vi "GetTextPositions.vi"(0 "reference":refnum<class "AbstractEdge.lvclass">, 1 "GraphicsRef":refnum<class "Graphics.lvclass">, 5 "error in (no error)":errorcluster) -> (14 "reference out":refnum<class "AbstractEdge.lvclass">, 15 "connectionPoints":T1[](array[typedef]) {"y" format="%.2f"; "x" format="%.2f"}, 19 "error out":errorcluster)   [LabVIEW 2014, in "AbstractEdge.lvclass"]
doc: "GetTextPositions"
uses:
  <resource>/Framework/Providers/Open_GDS/UML/AbstractEdge_class/AbstractEdge.lvclass
  <resource>/Framework/Providers/Open_GDS/UML/General/Point/Point Point2D.ctl
  <resource>/Framework/Providers/Open_GDS/UML/Graphics_class/Graphics.lvclass
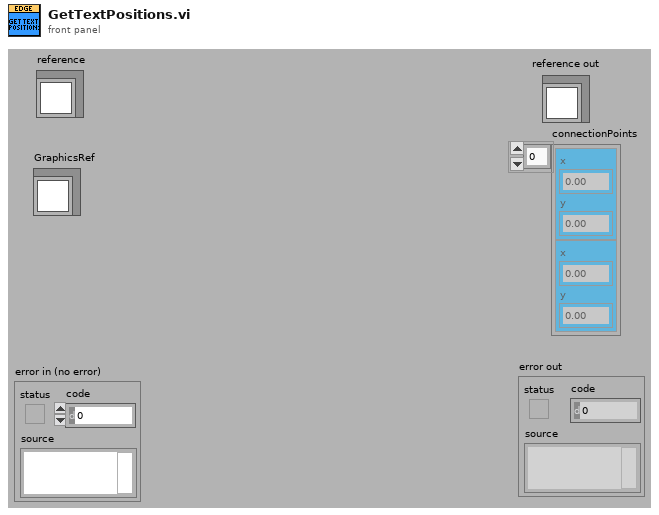
[diagram p1: front panel]
types:
  T1 = typedef "Point Point2D.ctl" = cluster{"x":dbl, "y":dbl}
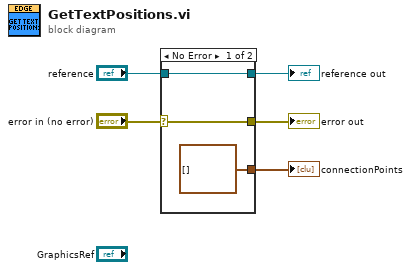
[diagram p0: block diagram]
diagram:
  n1 = case shown="No Error" "error in (no error)" {
    selector: "error in (no error)" -> [w7 w9]
    tunnel: "reference" -> [w8 w10]
    tunnel: [w7 w9] -> w4
    tunnel: [w8 w10] -> w3
    tunnel: [T1[] [] ("connectionPoints") _] -> w1
    frame No Error {
    }
    frame Error {
    }
  }
  "reference out" <- w3
  "error out" <- w4
  "connectionPoints" <- w1
